vi "spectrum analyzer.vi"() -> ()   [LabVIEW 2023]
uses:
  <vilib>/measure/matone.llb/Extract Single Tone Information N Chan.vi
  <vilib>/express/express analysis/Spectral/Block/exnSpectralBlock spectral measurements RMS poly.vi
  <vilib>/express/express analysis/Spectral/Block/exnSpectralBlock spectral measurements RMS DDT.vi
  <vilib>/express/express analysis/Spectral/XNode/ExpressSpectralMeasurementsBlockNode.xnode
  <vilib>/measure/NI_MAPro.lvlib
panel:
  out "Note":string
  out "Frequency":dbl[](array[numeric]) format="%.2p"
  in  "Duration (s)":dbl=1.0
  in  "stop":bool
  in  "Run":bool
  out "Waveform Graph":dynamicdata(graph)
  out "Data":dynamicdata(graph)
  # "Spectrum Analyzer"
  # "Stop"
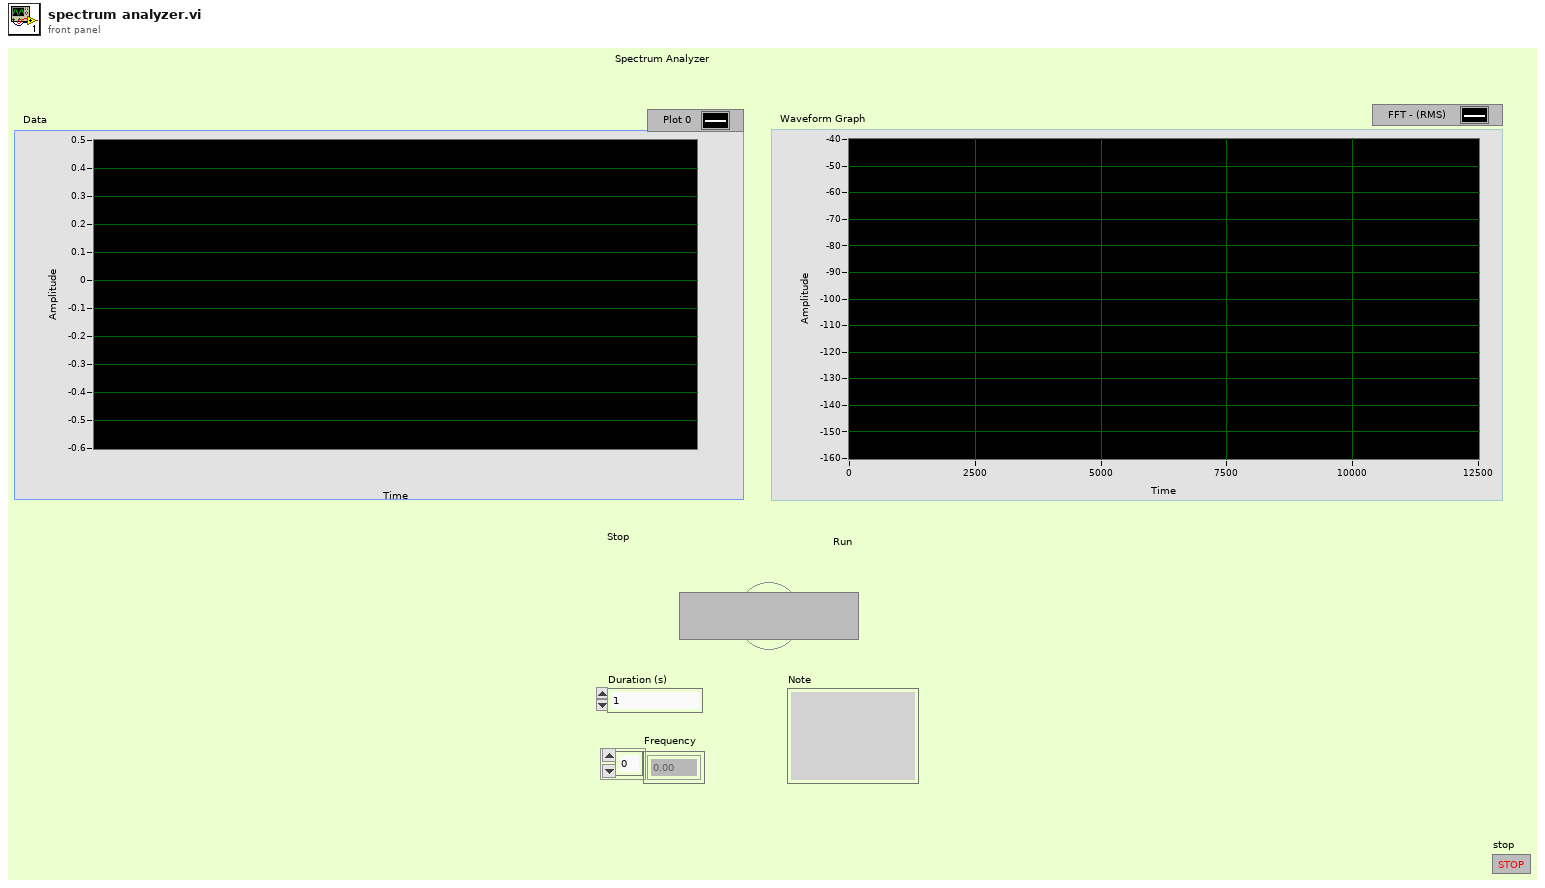
[diagram p1: front panel]
types:
  T1 = cluster{"averaging mode":u16, "weighting mode":u16, "number of averages":u32}
  T2 = cluster{"dB On (F)":bool, "unwrap phase (F)":bool, "convert to degree (F)":bool}
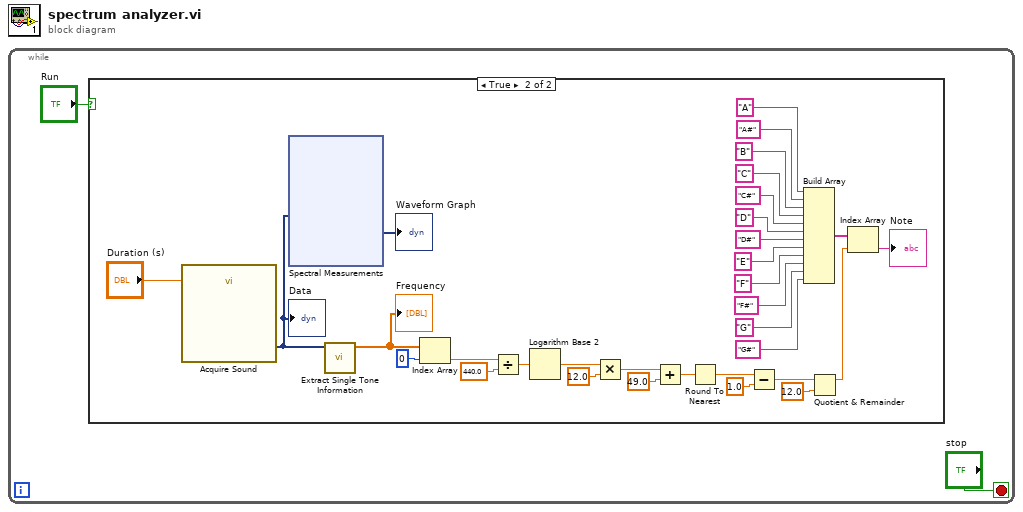
[diagram p0: block diagram]
diagram:
  n1 = while {
    stop <- "stop" stop-if-true
    n2 = case shown="True" "Run" {
      frame False {
      }
      frame True {
        n3 = call "Acquire Sound"("Duration (s)"="Duration (s)") -> ("Data"=w32:dynamicdata)  [unwired: 17 in, 1 out]
        "Data" <- w32
        n4 = xnode "Spectral Measurements"("Signals"=w32) -> ("FFT - (RMS)"=→"Waveform Graph":dynamicdata)  [unwired: 1 in, 2 out]
        n5 = call-poly <vilib>:"Extract Single Tone Information.vi"("time signals in"=w32) -> ("detected frequencies"=w6:dbl[])  [unwired: 5 in, 5 out]
        "Frequency" <- w6
        n6 = Index Array(array=w6, index=0) -> (element=w4:dbl)
        n7 = Divide(x=w4, y=440.0 ("detected frequency")) -> (x/y=w18:dbl)
        n8 = Logarithm Base 2(1:w18) -> (0:w17:dbl)
        n9 = Multiply(x=w17, y=12.0 ("detected frequency")) -> (x*y=w15:dbl)
        n10 = Add(x=w15, y=49.0 ("detected frequency")) -> (x+y=w13:dbl)
        n11 = Round To Nearest(number=w13) -> (nearest integer value=w12:dbl)
        n12 = Subtract(x=w12, y=1.0 ("detected frequency")) -> (x-y=w10:dbl)
        n13 = Build Array("A", "A#" ("element"), "B" ("element"), "C" ("element"), "C#" ("element"), "D" ("element"), "D#" ("element"), "E" ("element"), "F" ("element"), "F#" ("element"), "G" ("element"), "G#" ("element")) -> (w8:string[])
        n14 = Quotient & Remainder(x=w10, y=12.0 ("detected frequency")) -> (x-y*floor(x/y)=w7:dbl)  [unwired: 1 out]
        n15 = Index Array(array=w8, index=w7) -> (element=→"Note":string)
      }
    }
  }
